vi "addPathToRunFolder.vi"(8 "error in (no error)":errorcluster, 10 "Path":path, 11 "ExperimentRunner in":refnum<class "ExperimentRunner.lvclass">) -> (0 "error out":errorcluster, 3 "ExperimentRunner out":refnum<class "ExperimentRunner.lvclass">)   [LabVIEW 2009, in "Views.lvlib" / "ExperimentControl.lvlib" / "ExperimentRunner.lvclass"]
doc: "Add .xml paths to the path array. If user selects a folder it looks into the folder and find all .xml paths and adds them. It does this recursively for all subfolders."
uses:
  ExperimentRunner.lvclass
  ExperimentRunner.lvclass/ExperimentRunner.ctl
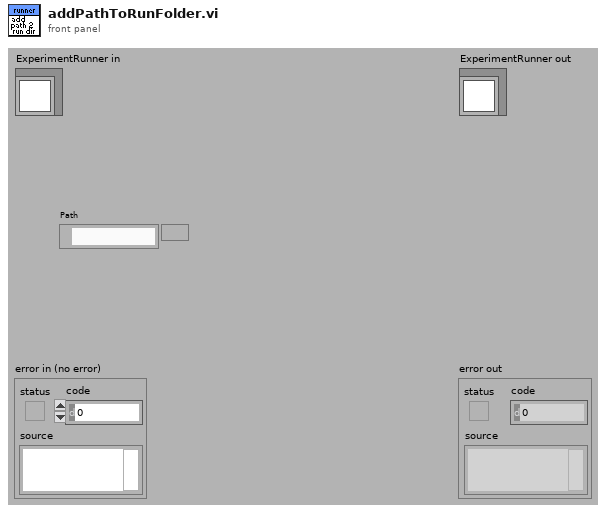
[diagram p1: front panel]
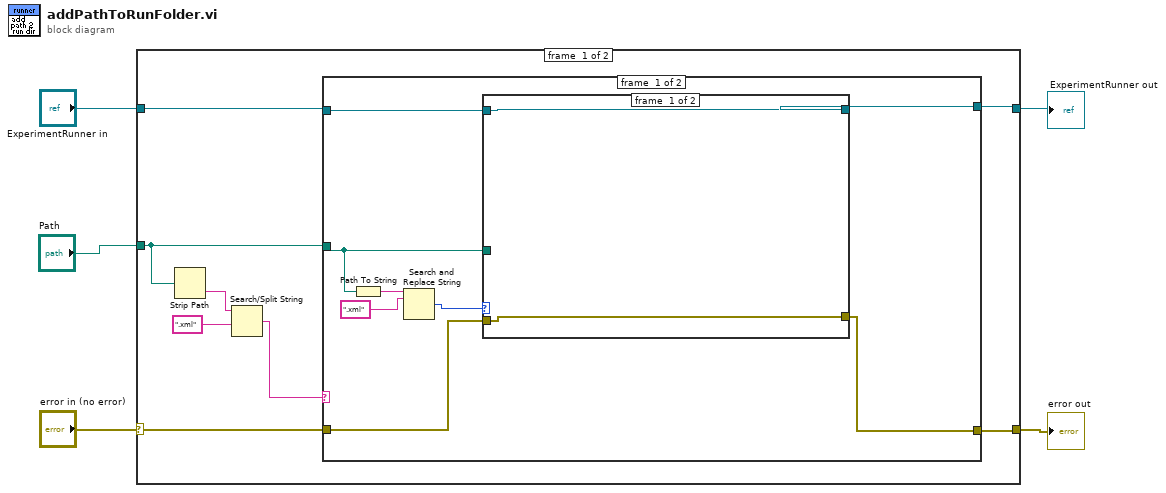
[diagram p0: block diagram]
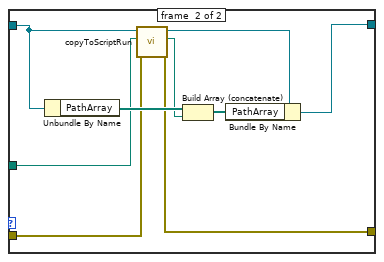
[diagram p2: hidden frame]
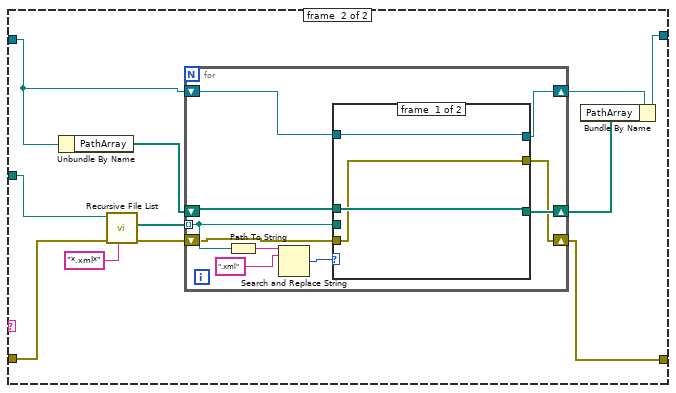
[diagram p3: hidden frame]
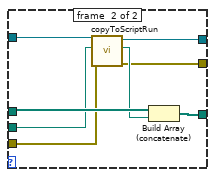
[diagram p4: hidden frame]
diagram:
  n1 = case shown="No Error" "error in (no error)" {
    selector: "error in (no error)" -> [w9 w66]
    tunnel: [w6 w66] -> w4
    tunnel: [w7 w65] -> w2
    tunnel: "ExperimentRunner in" -> [w8 w65]
    tunnel: "Path" -> [w10 _]
    frame #0 {
      n2 = Strip Path(path=w10) -> (name=w13:string)  [unwired: 1 out]
      n3 = Search/Split String(string=w13, search string/char (-)=".xml") -> (match + rest of string=w11:string)  [unwired: 1 in, 2 out]
      n4 = case shown="\"\"" w11 {
        tunnel: w10 -> [w19 w43]
        tunnel: w9 -> [w15 w41]
        tunnel: w8 -> [w21 w36]
        tunnel: [w14 w33] -> w6
        tunnel: [w20 w40] -> w7
        frame #0 {
          n5 = Path To String(path=w19) -> (string=w18:string)
          n6 = Search and Replace String(input string=w18, search string=".xml") -> (number of replacements=w16:i32)  [unwired: 6 in, 3 out]
          n7 = case shown="1, Default" w16 {
            tunnel: w21 -> [w23 w30]
            tunnel: [w23 w26] -> w20
            tunnel: w19 -> [_ w29]
            tunnel: w15 -> [w22 w25]
            tunnel: [w22 w24] -> w14
            frame #0 {
            }
            frame #1 {
              n8 = Unbundle By Name(w30) -> ("PathArray"=w32:path[])
              n9 = call "copyToScriptRun.vi"("error in (no error)"=w25, "Path"=w29, "ExperimentRunner in"=w30) -> ("error out"=w24:errorcluster, "Path out"=w28:path, "ExperimentRunner out"=w27:refnum<class "ExperimentRunner.lvclass">)  [unwired: 6 in]
              n10 = Build Array (concatenate)(w32, w28) -> (w31:path[])
              n11 = Bundle By Name(cluster=w27, "PathArray"=w31) -> (w26:refnum<class "ExperimentRunner.lvclass">)
            }
          }
        }
        frame #1 {
          n12 = Unbundle By Name(w36) -> ("PathArray"=w38:path[])
          n13 = call <vilib>:"Recursive File List.vi"("pattern"="*.xml*", "error in (no error)"=w41, "Folder Path"=w43) -> ("error out"=w34:errorcluster, "All Files in Dir"=w39:path[])  [unwired: 4 in, 3 out]
          n14 = for {
            tunnel: w39 -> [w49] mode=indexing
            shift-right: [w48] -> w37
            shift-left: w38 -> [w50]
            shift-right: [w46] -> w35
            shift-left: w36 -> [w47]
            shift-right: [w44] -> w33
            shift-left: w34 -> [w45]
            n15 = Path To String(path=w49) -> (string=w53:string)
            n16 = Search and Replace String(input string=w53, search string=".xml") -> (number of replacements=w51:i32)  [unwired: 6 in, 3 out]
            n17 = case shown="1, Default" w51 {
              tunnel: w50 -> [w56 w64]
              tunnel: w49 -> [_ w61]
              tunnel: [w56 w63] -> w48
              tunnel: w47 -> [w55 w62]
              tunnel: [w55 w59] -> w46
              tunnel: w45 -> [w54 w58]
              tunnel: [w54 w57] -> w44
              frame #0 {
              }
              frame #1 {
                n18 = call "copyToScriptRun.vi"("error in (no error)"=w58, "Path"=w61, "ExperimentRunner in"=w62) -> ("error out"=w57:errorcluster, "Path out"=w60:path, "ExperimentRunner out"=w59:refnum<class "ExperimentRunner.lvclass">)  [unwired: 6 in]
                n19 = Build Array (concatenate)(w64, w60) -> (w63:path[])
              }
            }
          }
          n20 = Bundle By Name(cluster=w35, "PathArray"=w37) -> (w40:refnum<class "ExperimentRunner.lvclass">)
        }
      }
    }
    frame #1 {
    }
  }
  "error out" <- w4
  "ExperimentRunner out" <- w2
